vi "AutoRocketHatch.vi"(10 "RightSideOfField?":bool, 11 "Coordinates":dbl[](array[numeric])) -> ()   [LabVIEW 2018]
uses:
  Globals.vi
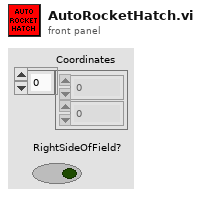
[diagram p1: front panel]
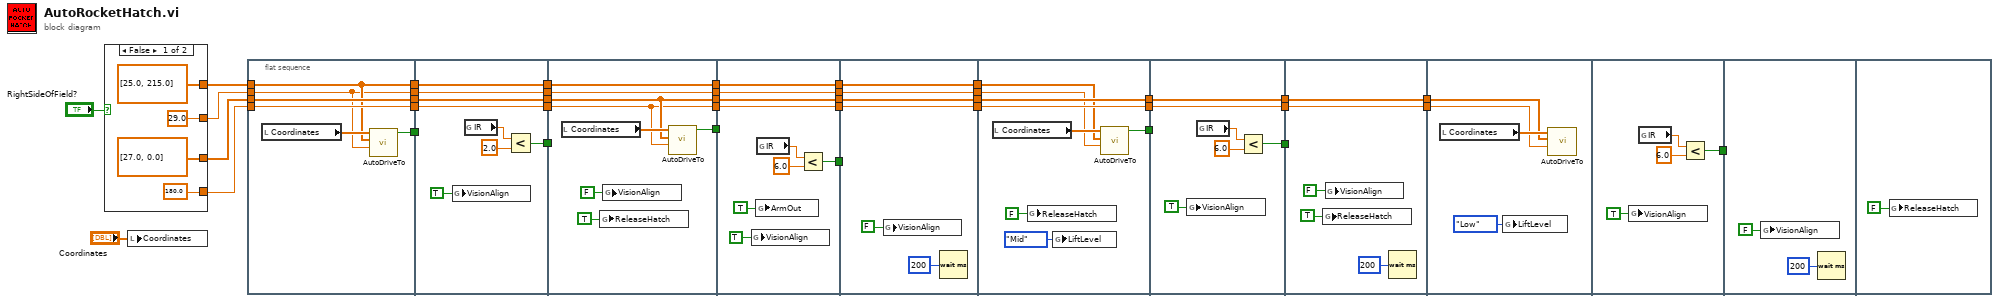
[diagram p0: block diagram]
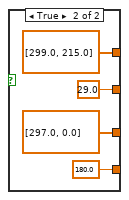
[diagram p2: hidden frame]
diagram:
  n1 = case shown="False" "RightSideOfField?" {
    tunnel: [dbl[] [27.0, 0.0] dbl[] [297.0, 0.0]] -> w36
    tunnel: [29.0 29.0] -> w37
    tunnel: [dbl[] [25.0, 215.0] dbl[] [299.0, 215.0]] -> w38
    tunnel: [180.0 180.0] -> w35
    frame False {
    }
    frame True {
    }
  }
  n2 = local write "Coordinates"("Coordinates") -> ()
  n3 = flat-sequence {
    tunnel: [w53] -> w33
    tunnel: w38 -> [w49]
    tunnel: w37 -> [w48]
    tunnel: w36 -> [w52]
    tunnel: w35 -> [w51]
    tunnel: [w52] -> w32
    tunnel: [w51] -> w31
    tunnel: [w49] -> w30
    tunnel: [w48] -> w29
    tunnel: [w58] -> w28
    tunnel: w33 -> [_]
    tunnel: w32 -> [w57]
    tunnel: w31 -> [w56]
    tunnel: [w57] -> w27
    tunnel: [w56] -> w26
    tunnel: [w55] -> w25
    tunnel: w30 -> [w55]
    tunnel: w29 -> [w54]
    tunnel: [w54] -> w24
    tunnel: w28 -> [_]
    tunnel: w27 -> [w65]
    tunnel: w26 -> [w64]
    tunnel: [w68] -> w11
    tunnel: [w67] -> w10
    tunnel: w25 -> [w67]
    tunnel: w24 -> [w66]
    tunnel: [w66] -> w8
    tunnel: [w65] -> w6
    tunnel: [w64] -> w4
    tunnel: w11 -> [_]
    tunnel: w10 -> [w78]
    tunnel: [w78] -> w9
    tunnel: w8 -> [w77]
    tunnel: [w77] -> w7
    tunnel: w6 -> [w76]
    tunnel: [w76] -> w5
    tunnel: w4 -> [w75]
    tunnel: [w75] -> w3
    tunnel: [w72] -> w2
    tunnel: [w84] -> w23
    tunnel: w9 -> [w84]
    tunnel: [w83] -> w22
    tunnel: w7 -> [w83]
    tunnel: [w82] -> w21
    tunnel: w5 -> [w82]
    tunnel: [w81] -> w20
    tunnel: w3 -> [w81]
    tunnel: w2 -> [_]
    tunnel: w23 -> [w88]
    tunnel: w22 -> [w87]
    tunnel: w21 -> [w92]
    tunnel: w20 -> [w91]
    tunnel: [w92] -> w19
    tunnel: [w91] -> w18
    tunnel: [w86] -> w17
    tunnel: w19 -> [w98]
    tunnel: w18 -> [w97]
    tunnel: [w98] -> w16
    tunnel: [w97] -> w15
    tunnel: [w93] -> w14
    tunnel: w17 -> [_]
    tunnel: w16 -> [w103]
    tunnel: w15 -> [w102]
    tunnel: w14 -> [_]
    tunnel: [w103] -> w13
    tunnel: [w102] -> w12
    tunnel: w13 -> [w106]
    tunnel: w12 -> [w105]
    tunnel: [w108] -> w1
    tunnel: w1 -> [_]
    frame #0 {
      n4 = local read "Coordinates"() -> (w50:dbl[])
      n5 = call "AutoDriveTo.vi"("EndAngle"=w48, "EndCoordinates"=w49, "Coordinates"=w50) -> ("ThereYet?"=w53:bool)  [unwired: 8 in]
    }
    frame #1 {
      n6 = global write "Globals.vi" "VisionAlign"(TRUE ("VisionAlign")) -> ()
      n7 = global read "Globals.vi" "IR"() -> (w60:dbl)
      n8 = Less?(x=w60, y=2.0) -> (x < y?=w58:bool)
    }
    frame #2 {
      n9 = local read "Coordinates"() -> (w69:dbl[])
      n10 = global write "Globals.vi" "ReleaseHatch"(TRUE ("ReleaseHatch")) -> ()
      n11 = global write "Globals.vi" "VisionAlign"(FALSE ("VisionAlign")) -> ()
      n12 = call "AutoDriveTo.vi"("EndAngle"=w64, "EndCoordinates"=w65, "Coordinates"=w69) -> ("ThereYet?"=w68:bool)  [unwired: 8 in]
    }
    frame #3 {
      n13 = global write "Globals.vi" "VisionAlign"(TRUE ("VisionAlign")) -> ()
      n14 = global write "Globals.vi" "ArmOut"(TRUE ("ArmOut")) -> ()
      n15 = global read "Globals.vi" "IR"() -> (w74:dbl)
      n16 = Less?(x=w74, y=6.0) -> (x < y?=w72:bool)
    }
    frame #4 {
      n17 = global write "Globals.vi" "VisionAlign"(FALSE ("VisionAlign")) -> ()
      n18 = Wait (ms)(milliseconds to wait=u32 200) -> ()  [unwired: 1 out]
    }
    frame #5 {
      n19 = local read "Coordinates"() -> (w89:dbl[])
      n20 = global write "Globals.vi" "ReleaseHatch"(FALSE ("ReleaseHatch")) -> ()
      n21 = global write "Globals.vi" "LiftLevel"(enum16{"Low", "Mid", "High"}."Mid" ("LiftLevel")) -> ()
      n22 = call "AutoDriveTo.vi"("EndAngle"=w87, "EndCoordinates"=w88, "Coordinates"=w89) -> ("ThereYet?"=w86:bool)  [unwired: 8 in]
    }
    frame #6 {
      n23 = global write "Globals.vi" "VisionAlign"(TRUE ("VisionAlign")) -> ()
      n24 = global read "Globals.vi" "IR"() -> (w95:dbl)
      n25 = Less?(x=w95, y=6.0) -> (x < y?=w93:bool)
    }
    frame #7 {
      n26 = global write "Globals.vi" "ReleaseHatch"(TRUE ("ReleaseHatch")) -> ()
      n27 = global write "Globals.vi" "VisionAlign"(FALSE ("VisionAlign")) -> ()
      n28 = Wait (ms)(milliseconds to wait=u32 200) -> ()  [unwired: 1 out]
    }
    frame #8 {
      n29 = local read "Coordinates"() -> (w107:dbl[])
      n30 = global write "Globals.vi" "LiftLevel"(enum16{"Low", "Mid", "High"}."Low" ("LiftLevel")) -> ()
      n31 = call "AutoDriveTo.vi"("EndAngle"=w105, "EndCoordinates"=w106, "Coordinates"=w107) -> ()  [unwired: 8 in, 1 out]
    }
    frame #9 {
      n32 = global write "Globals.vi" "VisionAlign"(TRUE ("VisionAlign")) -> ()
      n33 = global read "Globals.vi" "IR"() -> (w110:dbl)
      n34 = Less?(x=w110, y=6.0) -> (x < y?=w108:bool)
    }
    frame #10 {
      n35 = global write "Globals.vi" "VisionAlign"(FALSE ("VisionAlign")) -> ()
      n36 = Wait (ms)(milliseconds to wait=u32 200) -> ()  [unwired: 1 out]
    }
    frame #11 {
      n37 = global write "Globals.vi" "ReleaseHatch"(FALSE ("ReleaseHatch")) -> ()
    }
  }
